vi "Post_AuthenticationCode_Request.vi"(8 "error in (no error)":errorcluster, 11 "Asana in":refnum<class "Asana.lvclass">) -> (0 "error out":errorcluster, 3 "Asana out":refnum<class "Asana.lvclass">)   [LabVIEW 2016, in "Asana.lvclass"]
uses:
  Asana.lvclass
  Asana.lvclass/Asana.ctl
  <vilib>/httpClient/POSTBuffer.vi
  <vilib>/httpClient/LabVIEWHTTPClient.lvlib
  <vilib>/addons/_JKI.lib/Serialization/JSON/JKI JSON Serialization.lvlib
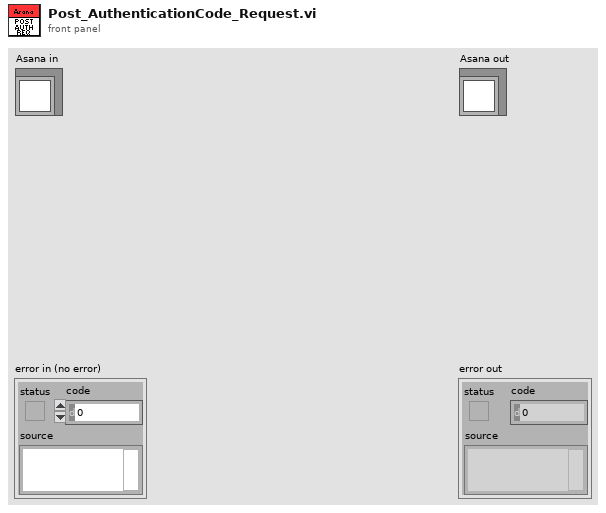
[diagram p1: front panel]
types:
  T1 = cluster{"token_type":string, "scope":string, "access_token":string, "refresh_token":string, "user_id":string, "expires_in":i32}
  T2 = typedef "LabVIEWHTTPClient.lvlib/ClientHandle.ctl" = refnum<k1>
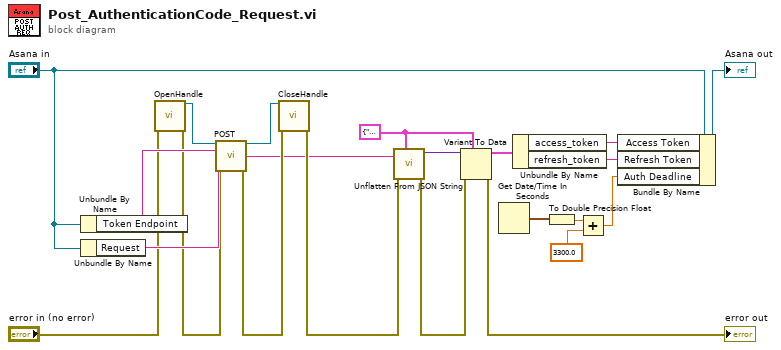
[diagram p0: block diagram]
diagram:
  w15 = T1 {"token_type"="", "scope"="", "access_token"="", "refresh_token"="", "user_id"="", "expires_in"=0}
  n1 = Unbundle By Name("Asana in") -> ("Token Endpoint"=w20:string)
  n2 = Unbundle By Name("Asana in") -> ("Request"=w19:string)
  n3 = call <vilib>:"OpenHandle.vi"("error in (no error)"="error in (no error)") -> ("client handle out"=w22:T2, "error out"=w17:errorcluster)  [unwired: 13 in]
  n4 = call-poly <vilib>:"POST.vi"("client handle"=w22, "url"=w20, "buffer"=w19, "error in (no error)"=w17) -> ("client handle out"=w21:T2, "body"=w1:string, "error out"=w16:errorcluster)  [unwired: 8 in, 1 out]
  n5 = call <vilib>:"CloseHandle.vi"("client handle"=w21, "error in (no error)"=w16) -> ("error out"=w9:errorcluster)  [unwired: 13 in]
  n6 = call <vilib>:"Unflatten From JSON String.vi"("Type and Defaults"=w15, "error in (no error)"=w9, "JSON String"=w1) -> ("error out"=w8:errorcluster, "Variant"=w14:variant)  [unwired: 7 in]
  n7 = Variant To Data(error in=w8, type=w15, Variant=w14) -> (data=w13:T1, error out=→"error out":errorcluster)
  n8 = Get Date/Time In Seconds() -> (seconds since 1Jan1904=w3:timestamp)
  n9 = Unbundle By Name(w13) -> ("access_token"=w12:string, "refresh_token"=w11:string)
  n10 = To Double Precision Float(number=w3) -> (double precision float=w4:dbl)
  n11 = Add(x=w4, y=3300.0) -> (x+y=w2:dbl)
  n12 = Bundle By Name(cluster="Asana in", "Access Token"=w12, "Refresh Token"=w11, "Auth Deadline"=w2) -> (→"Asana out":refnum<class "Asana.lvclass">)
